vi "命令入队列.vi"(8 "error in (no error)":errorcluster caption="错误输入（无错误）", 10 "命令类.lvclass":refnum<class "命令类.lvclass">, 11 "控制盒（队列） 输入":refnum<class "控制盒（队列）.lvclass"> caption="DNL_LabVIEW Object in") -> (0 "error out":errorcluster caption="错误输出", 3 "控制盒（队列） 输出":refnum<class "控制盒（队列）.lvclass"> caption="DNL_LabVIEW Object out")   [LabVIEW 2011, in "控制盒（队列）.lvclass"]
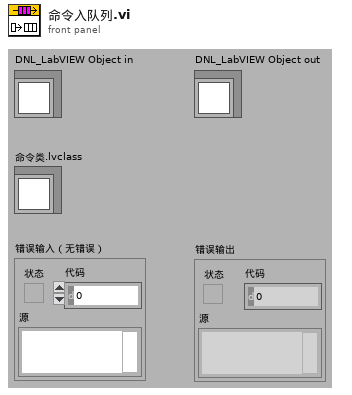
[diagram p1: front panel]
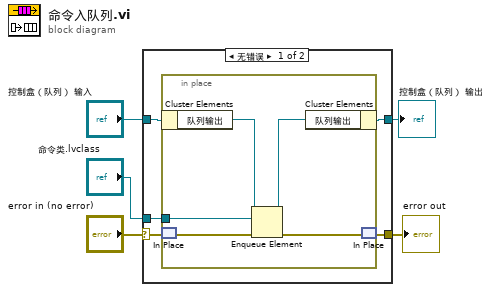
[diagram p0: block diagram]
diagram:
  n1 = case shown="无错误" "error in (no error)" {
    selector: "error in (no error)" -> [w8 w17]
    tunnel: [w7 w17] -> w4
    tunnel: [w6 w16] -> w2
    tunnel: "控制盒（队列） 输入" -> [w10 w16]
    tunnel: "命令类.lvclass" -> [w9 _]
    frame No Error {
      n2 = in-place {
        in-place-border: w9 -> [w13]
        n3 = in-place-cluster #1(w10) -> ("队列输出"=w15:refnum<queue>)
        n4 = in-place-match #2(w8) -> (w12:errorcluster)
        n5 = Enqueue Element(queue=w15, element=w13, error in (no error)=w12) -> (queue out=w14:refnum<queue>, error out=w11:errorcluster)  [unwired: 1 in, 1 out]
        n6 = in-place-cluster #1("队列输出"=w14) -> (w6:refnum<class "控制盒（队列）.lvclass">)
        n7 = in-place-match #2(w11) -> (w7:errorcluster)
      }
    }
    frame Error {
    }
  }
  "error out" <- w4
  "控制盒（队列） 输出" <- w2
